vi "Emi Cmd2.vi"(0 "X-CAN en entrée":refnum<class "X-CAN.lvclass">, 1 "Numéro Process [0..16] :":u8 max=16 step=1, 2 "Exploitation :":bool, 3 "Ack Piece :":bool, 4 "Crédit :":u8, 5 "entrée d'erreur (pas d'erreur)":errorcluster, 8 "Emission":bool) -> (14 "X-CAN en sortie":refnum<class "X-CAN.lvclass">, 19 "sortie d'erreur":errorcluster)   [LabVIEW 2014]
uses:
  <vilib>/Stratom, Inc/X-CAN for myRIO (API)/X-CAN Class/X-CAN.lvclass
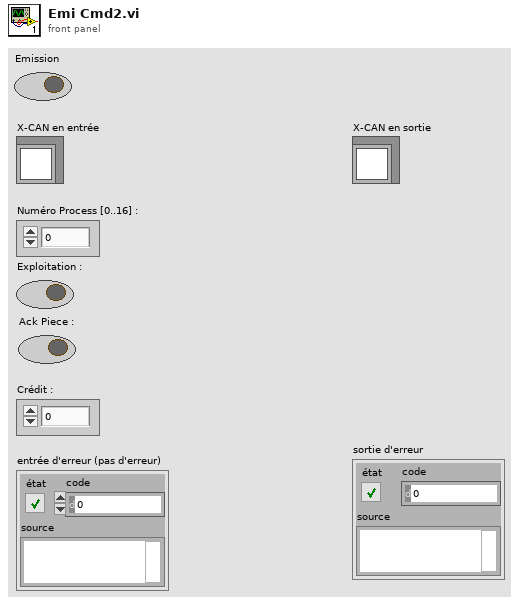
[diagram p1: front panel]
types:
  T1 = cluster{i32, bool, bool, u8[], "seconds since 1Jan1904":timestamp}
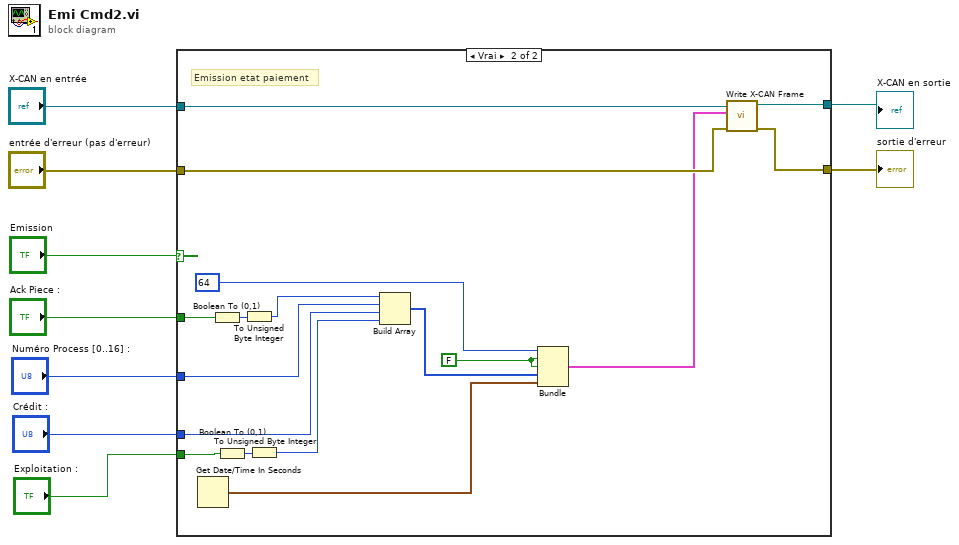
[diagram p0: block diagram]
diagram:
  n1 = case shown="Vrai" "Emission" {
    tunnel: [w10 w28] -> w9
    tunnel: "entrée d'erreur (pas d'erreur)" -> [w10 w27]
    tunnel: [w11 w26] -> w7
    tunnel: "X-CAN en entrée" -> [w11 w25]
    tunnel: "Ack Piece :" -> [_ w20]
    tunnel: "Numéro Process [0..16] :" -> [_ w19]
    tunnel: "Crédit :" -> [_ w16]
    tunnel: "Exploitation :" -> [_ w14]
    frame False {
    }
    frame True {
      w21 = FALSE
      # "Emission etat paiement"
      n2 = Get Date/Time In Seconds() -> (seconds since 1Jan1904=w24:timestamp)
      n3 = Boolean To (0,1)(Boolean=w20) -> (0, 1=w18:i16)
      n4 = Boolean To (0,1)(Boolean=w14) -> (0, 1=w15:i16)
      n5 = To Unsigned Byte Integer(number=w18) -> (unsigned 8bit integer=w17:u8)
      n6 = To Unsigned Byte Integer(number=w15) -> (unsigned 8bit integer=w13:u8)
      n7 = Build Array(w17, w19, w16, w13) -> (w22:u8[])
      n8 = Bundle(64, w21, w21, w22, "seconds since 1Jan1904"=w24) -> (w12:T1)  [unwired: 1 in]
      n9 = call <vilib>:"Write X-CAN Frame.vi"("error in"=w27, "CAN Frame"=w12, "X-CAN Session in"=w25) -> ("error out"=w28:errorcluster, "X-CAN Session out"=w26:refnum<class "X-CAN.lvclass">)  [unwired: 7 in]
    }
  }
  "sortie d'erreur" <- w9
  "X-CAN en sortie" <- w7
